vi "Export to Kepware Server.vi"(7 "selected path":path, 8 "error in":errorcluster, 11 "Device Ref in":T1 format="%.0x") -> (0 "error out":errorcluster)   [LabVIEW 2021]
uses:
  <vilib>/NI VeriStand/Custom Device API/Custom Device Item Ref.ctl
  Modbus Master System Explorer.lvlib
  <vilib>/NI VeriStand/Custom Device API/Custom Device API.lvlib
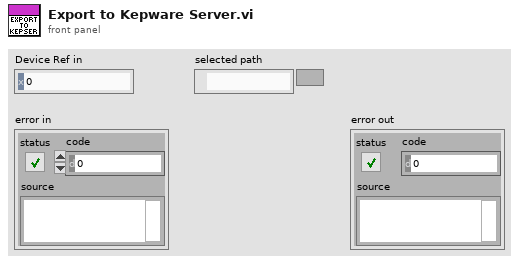
[diagram p1: front panel]
types:
  T1 = typedef "Custom Device API.lvlib/Custom Device Item Ref.ctl" = u64
  T2 = typedef "Modbus Master Shared.lvlib/Channel Data.ctl" = cluster{"Coils":T3[], "Discrete Inputs":T3[], "Input Registers":T3[], "Holding Registers":T3[]}
  T3 = typedef "Modbus Master Shared.lvlib/Channel.ctl" = cluster{"Name":string, "Modbus Type":T4, "Veristand Type":T5, "Mapping":T6}
  T4 = typedef "Modbus Master Shared.lvlib/Modbus Type.ctl" = enum16{"Coil", "Discrete Input", "Holding Register", "Input Register"}
  T5 = typedef "Custom Device API.lvlib/Custom Device Channel Type.ctl" = enum16{"Input", "Output"}
  T6 = typedef "Modbus Master Shared.lvlib/Mapping.ctl" = cluster{"DataType":T7, "Unit ID":u8, "Starting Address":u16, "Sub-Index (Bool)":u16, "VS Reference":T1}
  T7 = typedef "Modbus Master Shared.lvlib/DataType.ctl" = enum16{"Double", "Single", "I64", "I32", "I16", "I8", "U64", "U32", "U16", "U8", "Boolean"}
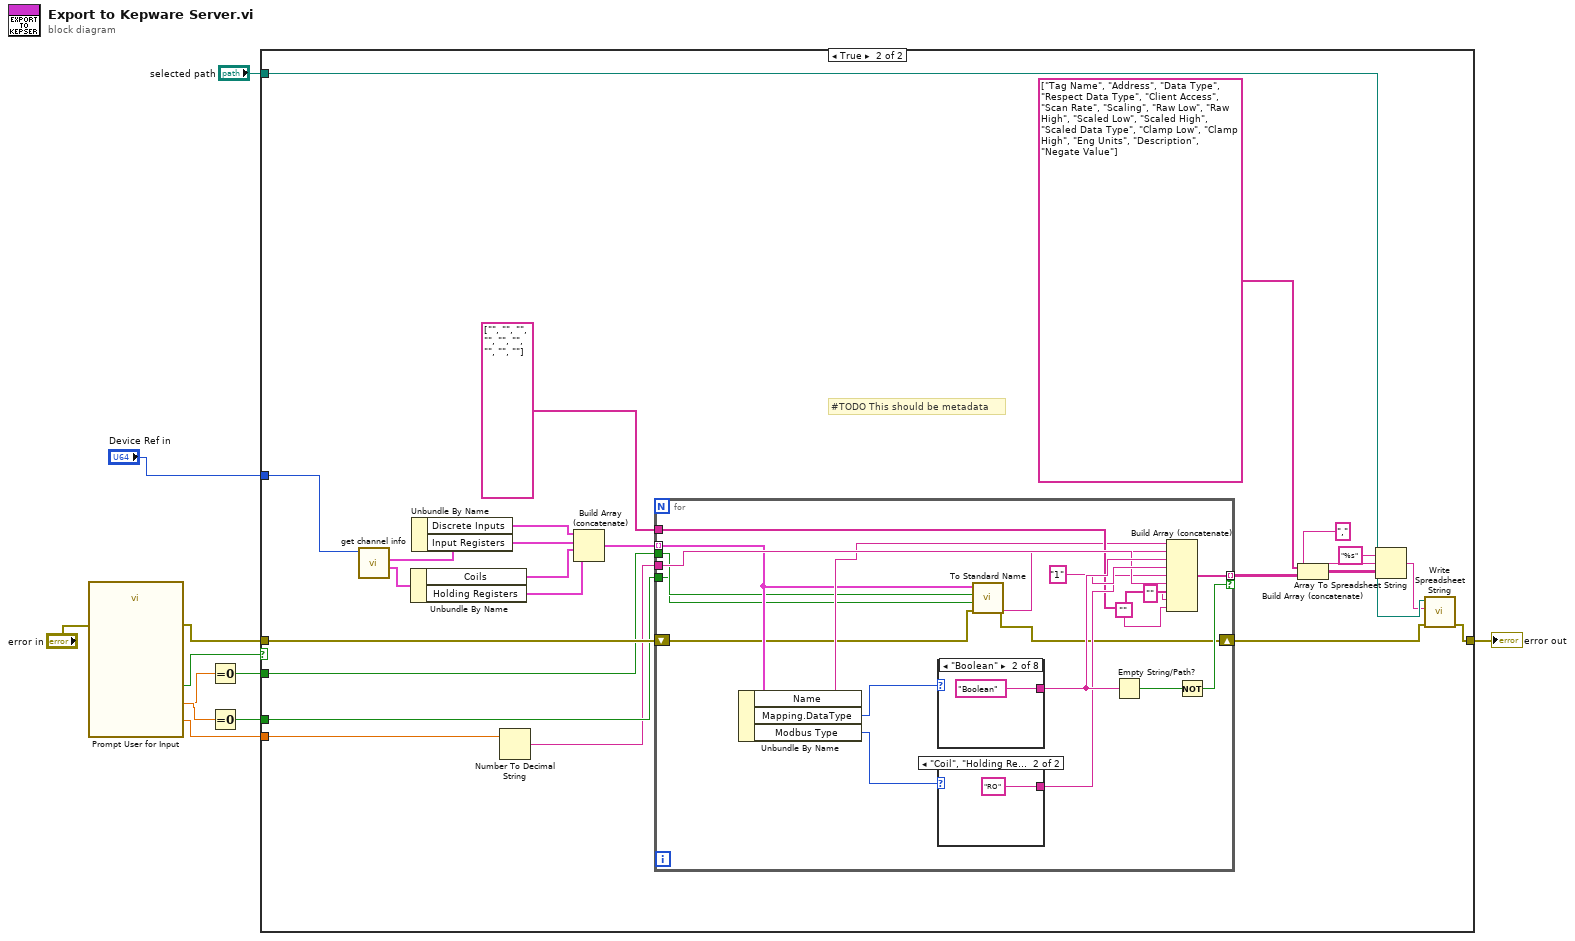
[diagram p0: block diagram]
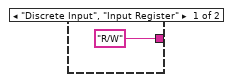
[diagram p3: hidden frame]
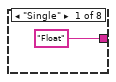
[diagram p4: hidden frame]
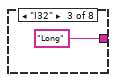
[diagram p5: hidden frame]
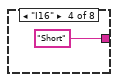
[diagram p6: hidden frame]
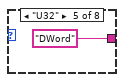
[diagram p7: hidden frame]
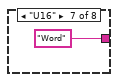
[diagram p9: hidden frame]
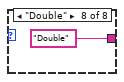
[diagram p10: hidden frame]
diagram:
  n1 = call "Prompt User for Input"("error in (no error)"="error in") -> ("Scan Rate (ms)"=w2:dbl, "Indexing for booleans (0 or 1)"=w6:dbl, "Indexing for register (0 or 1)"=w5:dbl, "OK"=w7:bool, "error out"=w8:errorcluster)  [unwired: 14 in]
  n2 = Equal To 0?(x=w5) -> (x = 0?=w4:bool)
  n3 = Equal To 0?(x=w6) -> (x = 0?=w3:bool)
  n4 = case shown="True" w7 {
    tunnel: "selected path" -> [_ w35]
    tunnel: [w12 w29] -> w10
    tunnel: w8 -> [w12 w28]
    tunnel: w4 -> [_ w27]
    tunnel: w3 -> [_ w26]
    tunnel: w2 -> [_ w23]
    tunnel: "Device Ref in" -> [_ w20]
    frame False {
    }
    frame True {
      # "#TODO This should be metadata"
      n5 = call "get channel info.vi"("Item Ref in"=w20) -> ("Outputs"=w18:T2, "Inputs"=w19:T2)  [unwired: 7 in, 2 out]
      n6 = Unbundle By Name(w18) -> ("Coils"=w15:T3[], "Holding Registers"=w14:T3[])
      n7 = Unbundle By Name(w19) -> ("Discrete Inputs"=w17:T3[], "Input Registers"=w16:T3[])
      n8 = Number To Decimal String(number=w23) -> (decimal integer string=w22:string)  [unwired: 1 in]
      n9 = Build Array (concatenate)(w17, w16, w15, w14) -> (w13:T3[])
      n10 = for {
        shift-right: [w38] -> w30
        shift-left: w28 -> [w39]
        tunnel: [w54] -> w33 mode=indexing if=w53
        tunnel: w27 -> [w41]
        tunnel: w26 -> [w40]
        tunnel: w22 -> [w48]
        tunnel: string[] ["", "", "", "", "", "", "", "", ""] ("array") -> [w46]
        tunnel: w13 -> [w42] mode=indexing
        n11 = Unbundle By Name(w42) -> ("Name"=w45:string, "Mapping.DataType"=w44:T7, "Modbus Type"=w43:T4)
        n12 = case shown="\"Boolean\"" w44 {
          tunnel: ["Float" "Boolean" "Long" "Short" "DWord" _ "Word" "Double"] -> w51
          frame "Single" {
          }
          frame "Boolean" {
          }
          frame "I32" {
          }
          frame "I16" {
          }
          frame "U32" {
          }
          frame Default {
          }
          frame "U16" {
          }
          frame "Double" {
          }
        }
        n13 = case shown="\"Coil\", \"Holding Register\"" w43 {
          tunnel: ["R/W" ("element") "RO" ("element")] -> w47
          frame "Discrete Input", "Input Register" {
          }
          frame "Coil", "Holding Register" {
          }
        }
        n14 = call "To Standard Name.vi"("error in (no error)"=w39, "zero index bit"=w40, "zero index element"=w41, "Channel"=w42) -> ("error out"=w38:errorcluster, "standard name"=w37:string)  [unwired: 6 in]
        n15 = Empty String/Path?(string/path=w51) -> (empty?=w52:bool)
        n16 = Build Array (concatenate)(w45, w37, w51, "1" ("element"), w47, w48, w46, "" ("element"), "") -> (w54:string[])
        n17 = Not(x=w52) -> (.not. x?=w53:bool)
      }
      n18 = Build Array (concatenate)(string[] ["Tag Name", "Address", "Data Type", "Respect Data Type", "Client Access", "Scan Rate", "Scaling", "Raw Low", "Raw High", "Scaled Low", "Scaled High", "Scaled Data Type", "Clamp Low", "Clamp High", "Eng Units", "Description", "Negate Value"] ("array"), w33) -> (w25:string[][])
      n19 = Array To Spreadsheet String(delimiter (Tab)="," ("delimiter (\\t)"), array=w25, 3:"%s" ("format (%s)")) -> (spreadsheet string=w31:string)
      n20 = call <vilib>:"Write Spreadsheet String.vi"("error in"=w30, "spreadsheet string"=w31, "file path (dialog if empty)"=w35) -> ("error out"=w29:errorcluster)  [unwired: 7 in, 1 out]
    }
  }
  "error out" <- w10
